vi "Test2_6.vi"(7 "Report Enable":bool, 8 "error in":errorcluster, 9 "Cycles Burst":i32=10000, 10 "DT_50_L0":i32[][](array[numeric]), 11 "Instrument VISA in":T1={"AWG VISA"="81160A", "Oscilloscope  VISA "="DSO80204B", "Integration Board IP"="172.16.7.43", "connection ID"=refnum, "report out"=refnum}) -> (0 "error out":errorcluster, 2 "Result":dbl[][][](array[numeric]), 3 "Instrument VISA out":T1={"AWG VISA"="81160A", "Oscilloscope  VISA "="DSO80204B", "Integration Board IP"="172.16.7.43", "connection ID"=refnum, "report out"=refnum})   [LabVIEW 2009]
uses:
  <vilib>/Analysis/NI_AALPro.lvlib
  <instrlib>/Agilent 81150/Agilent 81150.lvlib
  <vilib>/Utility/NIReport.llb/NI_report.lvclass
panel:
  out "XY Graph":cluster{"Y":dbl[], "Y":dbl[]}[](graph)
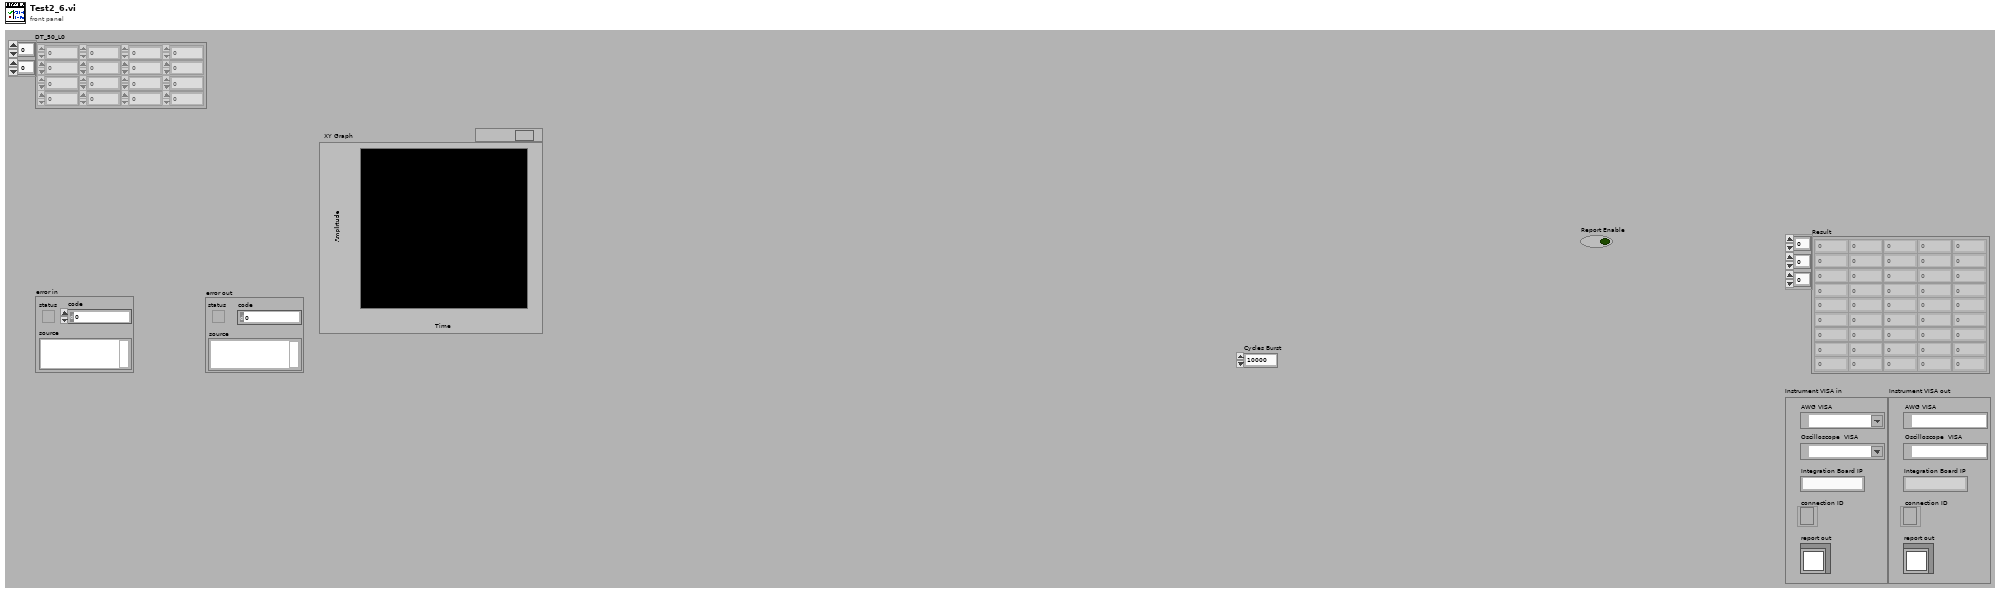
[diagram p1: front panel]
types:
  T1 = cluster{"AWG VISA":refnum<visa-resource-name>, "Oscilloscope  VISA ":refnum<visa-resource-name>, "Integration Board IP":string, "connection ID":refnum<k5>, "report out":refnum<class "NI_report.lvclass">}
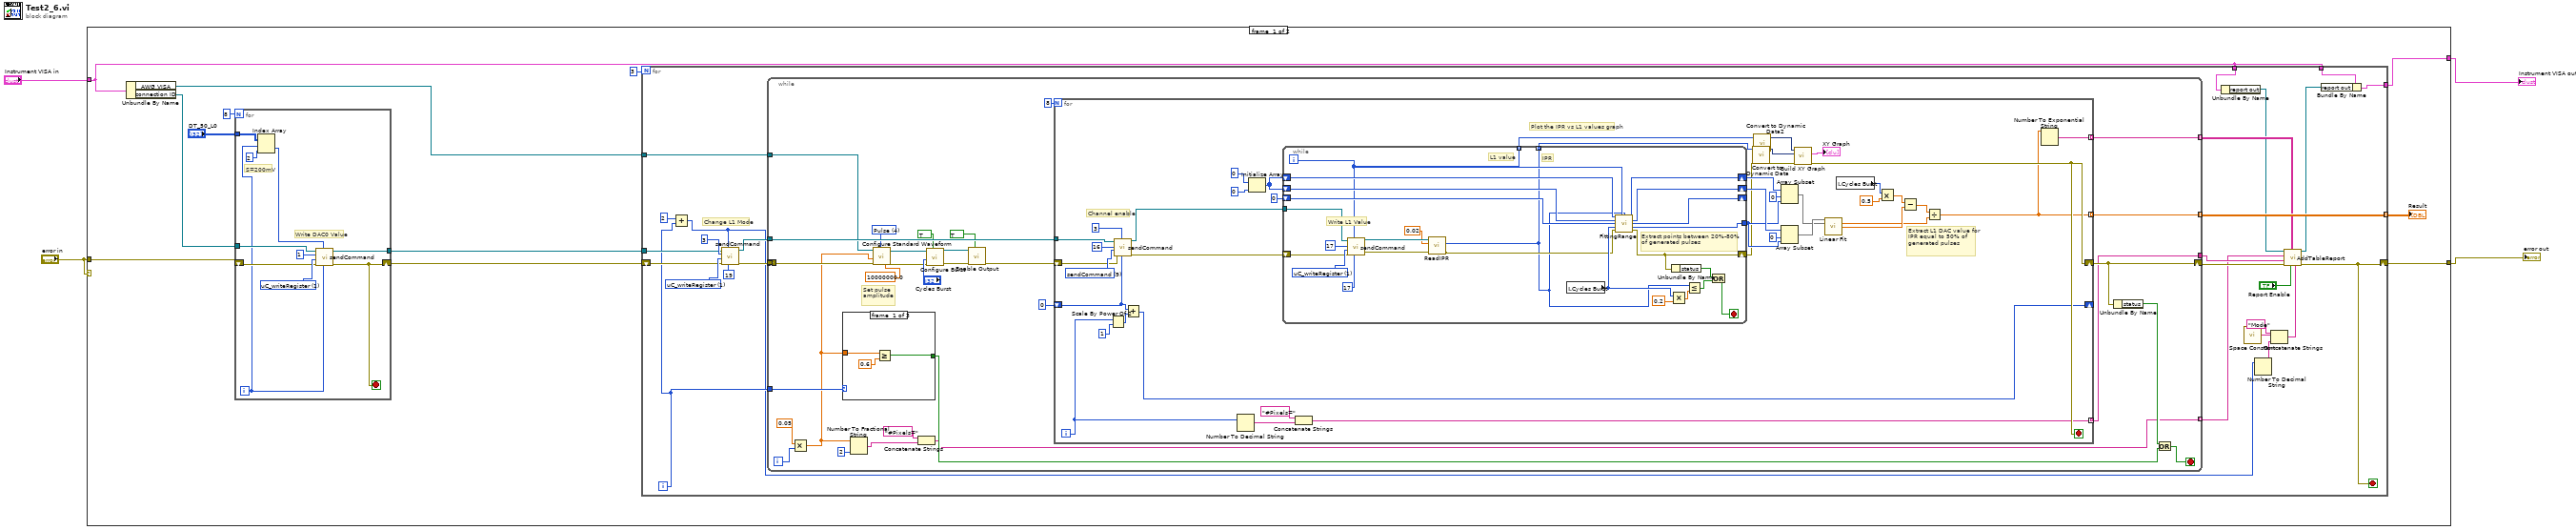
[diagram p0: block diagram]
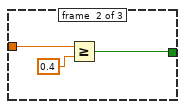
[diagram p2: hidden frame]
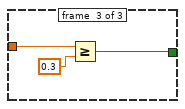
[diagram p3: hidden frame]
diagram:
  n1 = case shown="No Error" "error in" {
    tunnel: "error in" -> [w13 w160]
    tunnel: "Instrument VISA in" -> [w6 w159]
    tunnel: [w11 w160] -> w3
    tunnel: [w5 w159] -> w1
    frame #0 {
      n2 = Unbundle By Name(w6) -> ("AWG VISA"=w8:refnum<visa-resource-name>, "connection ID"=w14:refnum<k5>)
      n3 = for {
        N: 8 -> [_]
        shift-right: [w149] -> w9
        shift-left: w13 -> [w155]
        tunnel: w14 -> [w153]
        tunnel: "DT_50_L0" -> [w156]
        tunnel: [w150] -> w10
        i -> [w151]
        stop <- w149 stop-if-true
        w158 = u16 1 items=["sendCommand"=9, "FPGA_writeRegister"=3, "FPGA_readRegister"=2, "uC_writeRegister"=1, "uC_readRegister"=0] ("Action")
        # "S=200mV"
        # "Write DAC0 Value"
        n4 = Index Array(array=w156, index (row)=w151, index (col)=2 ("disabled index (col)")) -> (element=w154:i32)
        n5 = call "sendCommand.vi"("Address"=w151, "Data"=w154, "error in"=w155, "Action"=w158, "id_in"=1 ("id"), "connection ID"=w153) -> ("error out"=w149:errorcluster, "connection ID out"=w150:refnum<k5>)  [unwired: 1 in, 3 out]
      }
      n6 = for {
        N: 3 -> [_]
        tunnel: [w39] -> w7 mode=indexing
        shift-right: [w31] -> w11
        shift-left: w9 -> [w38]
        tunnel: w10 -> [w37]
        tunnel: w8 -> [w34]
        tunnel: w6 -> [w28]
        tunnel: w6 -> [w26]
        tunnel: [w25] -> w5
        i -> [w33]
        stop <- w31 stop-if-true
        w43 = u16 1 items=["sendCommand"=9, "FPGA_writeRegister"=3, "FPGA_readRegister"=2, "uC_writeRegister"=1, "uC_readRegister"=0] ("Action")
        # "Change L1 Mode"
        n7 = Add(x=2, y=w33) -> (x+y=w20:i32)
        n8 = call "sendCommand.vi"("Address"=19, "Data"=w20, "error in"=w38, "Action"=w43, "id_in"=3 ("id"), "connection ID"=w37) -> ("error out"=w35:errorcluster, "connection ID out"=w40:refnum<k5>)  [unwired: 1 in, 3 out]
        n9 = while {
          tunnel: w40 -> [w71]
          tunnel: [w70] -> w39 mode=indexing
          tunnel: w35 -> [w60]
          tunnel: w34 -> [w58]
          tunnel: w33 -> [w55]
          shift-right: [w54] -> w32
          shift-left: _ -> [_]
          tunnel: [w50] -> w29 mode=indexing
          tunnel: [w45] -> w17 mode=indexing
          tunnel: [w44] -> w18
          i -> [w57]
          stop <- w51 stop-if-true
          w68 = u16 4 items=["Sine", "Square", "Ramp Up", "Ramp Down", "Pulse", "Noise", "DC"] ("Waveform (0: Sine)")
          # "Set pulse amplitude"
          n10 = Multiply(x=0.05, y=w57) -> (x*y=w47:dbl)
          n11 = case shown="0, Default" w55 {
            tunnel: w47 -> [w76 w78 w82]
            tunnel: [w74 w77 w80] -> w52
            frame #0 {
              n12 = Greater Or Equal?(x=w76, y=0.6) -> (x >= y?=w74:bool)
            }
            frame #1 {
              n13 = Greater Or Equal?(x=w78, y=0.4) -> (x >= y?=w77:bool)
            }
            frame #2 {
              n14 = Greater Or Equal?(x=w82, y=0.3) -> (x >= y?=w80:bool)
            }
          }
          n15 = Number To Fractional String(number=w47, precision (6)=i16 2) -> (F-format string=w48:string)  [unwired: 2 in]
          n16 = call <instrlib>:"Configure Standard Waveform.vi"("Frequency (1000.0 Hz)"=10000000.0, "Waveform (0: Sine)"=w68, "error in (no error)"=w60, "Amplitude (1.0 Vpp)"=w47, "VISA resource name"=w58) -> ("error out"=w62:errorcluster, "VISA resource name out"=w61:refnum<visa-resource-name>)  [unwired: 5 in]
          n17 = Concatenate Strings("#Pixels=" ("string"), w48) -> (w45:string)
          n18 = call <instrlib>:"Configure Burst.vi"("Enable Burst (F: Disable)"=TRUE, "error in (no error)"=w62, "Burst Count (2)"="Cycles Burst", "VISA resource name"=w61) -> ("error out"=w65:errorcluster, "VISA resource name out"=w64:refnum<visa-resource-name>)  [unwired: 6 in]
          n19 = call <instrlib>:"Enable Output.vi"("Enable Output (T: Enable)"=TRUE, "error in (no error)"=w65, "VISA resource name"=w64) -> ("error out"=w59:errorcluster)  [unwired: 7 in, 1 out]
          n20 = for {
            N: 8 -> [_]
            tunnel: [w88] -> w70 mode=indexing
            shift-right: [w117] -> w54
            shift-left: w59 -> [w120]
            shift-right: [w113] -> _
            shift-left: 0 ("x") -> [w114]
            tunnel: w71 -> [w112]
            tunnel: [w87] -> w50 mode=indexing
            tunnel: [w83] -> w44 mode=indexing
            i -> [w84]
            stop <- w117 stop-if-true
            w123 = u16 9 items=["sendCommand"=9, "FPGA_writeRegister"=3, "FPGA_readRegister"=2, "uC_writeRegister"=1, "uC_readRegister"=0] ("Action")
            # "Extract L1 DAC value for IPR equal to 50% of generated pulses"
            # "Plot the IPR vs L1 values graph"
            # "Channel enable"
            n21 = Scale By Power Of 2(n=w84, x=1) -> (x*2^n=w115:i32)
            n22 = call "sendCommand.vi"("Address"=w114, "Data"=3, "error in"=w120, "Action"=w123, "id_in"=16 ("id"), "connection ID"=w112) -> ("error out"=w118:errorcluster, "connection ID out"=w116:refnum<k5>)  [unwired: 1 in, 3 out]
            n23 = Add(x=w114, y=w115) -> (x+y=w113:i32)
            n24 = Number To Decimal String(number=w84) -> (decimal integer string=w86:string)  [unwired: 1 in]
            n25 = Initialize Array(0 ("element"), 0 ("dimension size")) -> (w104:i32[])
            n26 = while {
              tunnel: [w124] -> w110 mode=indexing
              tunnel: [w136] -> w108 mode=indexing
              shift-right: [w143] -> w102
              shift-left: w104 -> [w141]
              shift-right: [w142] -> w101
              shift-left: w104 -> [w140]
              shift-right: [w132] -> w89
              shift-left: w118 -> [w146]
              shift-right: [w138] -> _
              shift-left: 0 ("Array Pointer out") -> [w139]
              tunnel: [w137] -> w98
              tunnel: w116 -> [w134]
              i -> [w136]
              stop <- w130 stop-if-true
              w148 = u16 1 items=["sendCommand"=9, "FPGA_writeRegister"=3, "FPGA_readRegister"=2, "uC_writeRegister"=1, "uC_readRegister"=0] ("Action")
              # "Extract points between 20%-80% of generated pulses"
              # "Write L1 Value"
              # "IPR"
              # "L1 value"
              n27 = call "sendCommand.vi"("Address"=17, "Data"=w136, "error in"=w146, "Action"=w148, "id_in"=17 ("id"), "connection ID"=w134) -> ("error out"=w128:errorcluster, "connection ID out"=w126:refnum<k5>)  [unwired: 1 in, 3 out]
              n28 = call "ReadIPR.vi"("error in"=w128, 10:0.02 ("Delay Time (s)"), "connection ID"=w126) -> ("error out"=w127:errorcluster, "IPR value"=w124:i32)  [unwired: 6 in, 1 out]
              n29 = local read "Cycles Burst"() -> (w135:i32)
              n30 = call "FittingRange.vi"("Array in (X)"=w141, "L0 DAC"=w136, "IPR"=w124, "Array in (Y)"=w140, "Array Pointer in"=w139, "Cycles Burst"=w135, "error in"=w127) -> ("Array out (X)"=w143:i32[], "Array out (Y)"=w142:i32[], "Array Pointer out"=w138:i32, "N_Array Elements"=w137:i32, "error out"=w132:errorcluster)  [unwired: 4 in]
              n31 = Multiply(x=w135, y=0.2) -> (x*y=w144:dbl)
              n32 = Unbundle By Name(w132) -> ("status"=w131:bool)
              n33 = Less Or Equal?(x=w124, y=w144) -> (x <= y?=w133:bool)
              n34 = Or(x=w131, y=w133) -> (x .or. y?=w130:bool)
            }
            n35 = Concatenate Strings("#Pixels=" ("string"), w86) -> (w83:string)
            n36 = call "Convert to Dynamic Data"("Array"=w110) -> ("Dynamic Data Type"=w109:dynamicdata)  [unwired: 3 in]
            n37 = call "Convert to Dynamic Data2"("Array"=w108) -> ("Dynamic Data Type"=w107:dynamicdata)  [unwired: 3 in]
            n38 = Array Subset(array=w101, index=0, length=w98) -> (w97:i32[])
            n39 = Array Subset(array=w102, index=0, length=w98) -> (w96:i32[])
            n40 = call "Build XY Graph"("error in (no error)"=w89, "Y Input"=w109, "X Input"=w107) -> ("error out"=w117:errorcluster, "XY Graph"=→"XY Graph":cluster{"Y":dbl[], "Y":dbl[]}[])  [unwired: 7 in]
            n41 = call <vilib>:"Linear Fit.vi"("Y"=w97, "X"=w96) -> ("slope"=w90:dbl, "intercept"=w92:dbl)  [unwired: 9 in, 3 out]
            n42 = local read "Cycles Burst"() -> (w95:i32)
            n43 = Multiply(x=w95, y=0.5) -> (x*y=w93:dbl)
            n44 = Subtract(x=w93, y=w92) -> (x-y=w91:dbl)
            n45 = Divide(x=w91, y=w90) -> (x/y=w88:dbl)
            n46 = Number To Exponential String(number=w88) -> (E-format string=w87:string)  [unwired: 3 in]
          }
          n47 = Unbundle By Name(w54) -> ("status"=w53:bool)
          n48 = Or(x=w53, y=w52) -> (x .or. y?=w51:bool)
        }
        n49 = Unbundle By Name(w28) -> ("report out"=w27:refnum<class "NI_report.lvclass">)
        n50 = call <vilib>:"Space Constant.vi"() -> ("String"=w22:string)
        n51 = Number To Decimal String(number=w20) -> (decimal integer string=w21:string)  [unwired: 1 in]
        n52 = Concatenate Strings("Mode" ("string"), w22, w21) -> (w19:string)
        n53 = call "AddTableReport.vi"("Table title"=w19, "Report Enable"="Report Enable", "Data"=w29, "error in"=w32, "Columns"=w18, "Rows"=w17, "report in"=w27) -> ("error out"=w31:errorcluster, "report out"=w24:refnum<class "NI_report.lvclass">)  [unwired: 3 in]
        n54 = Bundle By Name(cluster=w26, "report out"=w24) -> (w25:T1)
      }
      "Result" <- w7
    }
    frame #1 {
    }
  }
  "error out" <- w3
  "Instrument VISA out" <- w1
